vi "Set Page.vi"(8 "Error In":errorcluster, 10 "Tab Control":refnum<vi>, 11 "Application In":refnum<class "Application.lvclass">) -> (0 "Error Out":errorcluster, 3 "Application Out":refnum<class "Application.lvclass">)   [LabVIEW 2019, in "Application.lvclass"]
doc: "The VI sets the page of the tab control whose reference is given."
uses:
  Application.lvclass
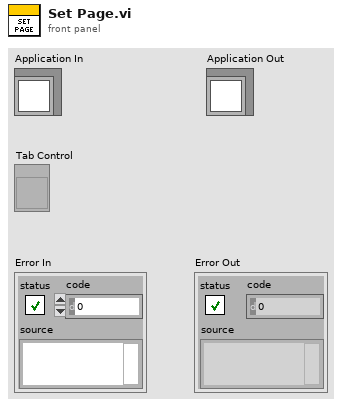
[diagram p1: front panel]
types:
  T1 = enum32{"Home Page", "Mode Page", "Configuration Page", "Input Page", "Result Page"}
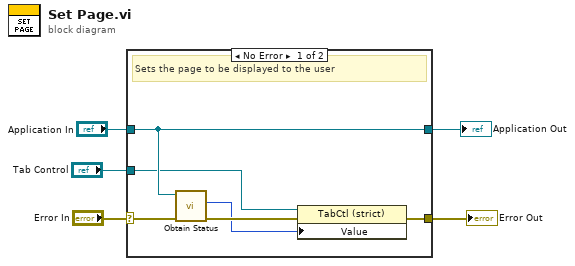
[diagram p0: block diagram]
diagram:
  n1 = case shown="No Error" "Error In" {
    selector: "Error In" -> [w11 w13]
    tunnel: [w8 w13] -> w4
    tunnel: "Tab Control" -> [w7 _]
    tunnel: "Application In" -> [w9 w12]
    tunnel: [w9 w12] -> w1
    frame No Error {
      # "Sets the page to be displayed to the user"
      n2 = call-dynamic "Obtain Status.vi"("Error In"=w11, "Application In"=w9) -> ("Error Out"=w10:errorcluster, "Page"=w6:T1)  [unwired: 6 in, 2 out]
      n3 = property class="TabCtl (strict)"(reference=w7, error in=w10, "Value"=w6) -> (error out=w8:errorcluster)  [unwired: 1 out]
    }
    frame Error {
    }
  }
  "Error Out" <- w4
  "Application Out" <- w1
